vi "T7 CheckLength KAG.vi"(0 "Array":u8[](array[numeric])=[139, 242, 0, 160, 247, 0]) -> (1 "Array Output":u8[](array[numeric])=[139, 242, 0, 160, 247, 0], 2 "CheckLength Error":bool)   [LabVIEW 2015]
doc: "The LabJack T7 MODBUS Feedback Auto-Reponse Packet Protocol includes 2 Parameters that can be used to check packet integrity: (1) Length : # of bytes after \"Length\" parameter, (2) Number of samples. Though slightly redundant, one could also check the for the expected size of the entire Packet Byte Array. If any of the expected parameter values is not equal to the calculated length value, the CheckLength Error = TRUE.\n\n~~~~~~~~~~~~~~~~~~~~~~~~~~~~~~~~~~~\nMore Details:\n\nTransaction ID: The device echos this value. Use to match responses with commands.\nProtocol ID: Not used. Just pass 0.\nLength: The number of bytes after the \"Length\" parameter, per the Modbus spec.\nUnit ID: Not used. Pass 1 to fit with convention.\nFunctionn #: 3 (Read Multiple), 4 (Read One), 6 (Write One), 16 (Write Multiple) are standard Modbus \"holding\" functions. 76 (Feedback -- Multiple Reads & Writes in a single packet) is LJ custom MBFB function."
panel:
  out "Calculated # Bytes":i32
  out "Input # Bytes":i32
  out "Calculated # Samples":i32
  out "Input # Samples":i32
  out "Calculated Length":i32
  out "Input Length":i32
  # "Transaction ID"
  # "Protocol ID"
  # "MSB"
  # "Length"
  # "LSB"
  # "1 (Unit ID)"
  # "76 (Function)"
  # "MSB"
  # "# Samples"
  # "LSB"
  # "Backlog"
  # "Status Code"
  # "Additional Status Info"
  # "Stream Data"
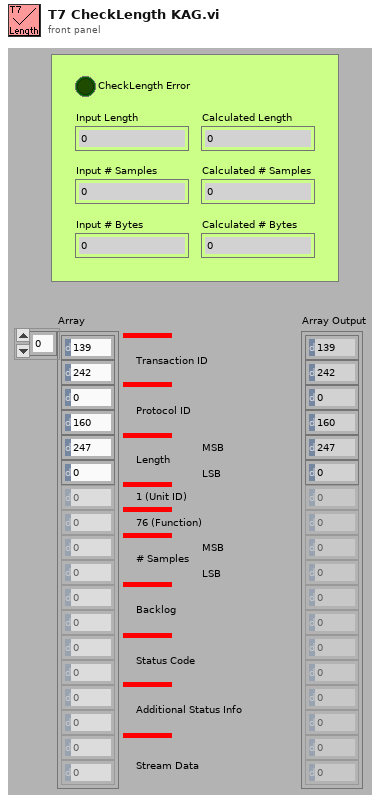
[diagram p1: front panel]
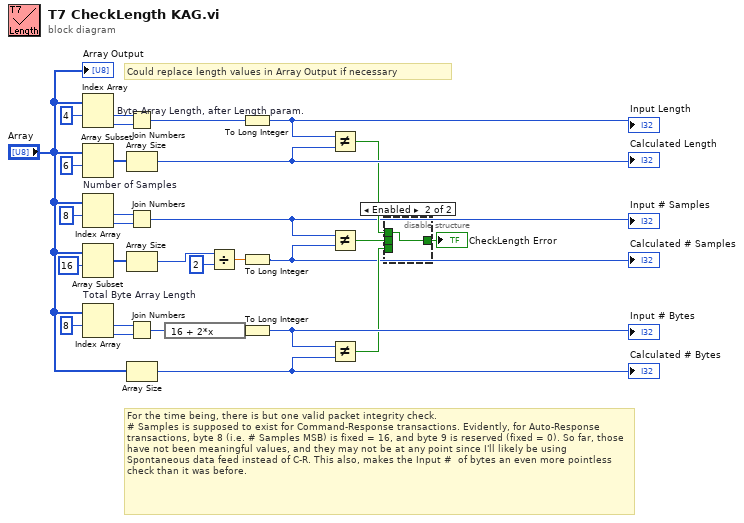
[diagram p0: block diagram]
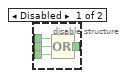
[diagram p2: hidden frame]
diagram:
  # "For the time being, there is but one valid packet integrity check.\n# Samples is supposed to exist for Command-Response transactions. Evidently, for Auto-Response transactions, byte 8 (i.e. # Samples MSB) is fixed = 16, and byte 9 is reserved (fixed = 0). So far, those have not been meaningful values, and they may not be at any point since I'll likely be using Spontaneous data feed instead of C-R. This also, makes the Input #  of bytes an even more pointless check than it was before."
  # "Could replace length values in Array Output if necessary"
  n1 = Index Array "Byte Array Length, after Length param."(array="Array", index #1=4 ("Index")) -> (element #1=w26:u8, element #2=w22:u8)  [unwired: 1 in]
  n2 = Array Subset(array="Array", index=6 ("Array Index")) -> (w27:u8[])  [unwired: 1 in]
  n3 = Index Array "Number of Samples"(array="Array", index #1=8 ("index")) -> (element #1=w21:u8, element #2=w20:u8)  [unwired: 1 in]
  n4 = Array Subset(array="Array", index=16 ("Array Index")) -> (w19:u8[])  [unwired: 1 in]
  n5 = Index Array "Total Byte Array Length"(array="Array", index #1=8 ("Index")) -> (element #1=w14:u8, element #2=w15:u8)  [unwired: 1 in]
  n6 = Join Numbers(hi=w26, lo=w22) -> ((hi.lo)=w25:u16)
  n7 = Array Size(array=w27) -> (size(s)=w24:i32)
  "Calculated Length" <- w24
  n8 = Join Numbers(hi=w21, lo=w20) -> ((hi.lo)=w1:u16)
  "Input # Samples" <- w1
  n9 = Array Size(array=w19) -> (size(s)=w3:i32)
  n10 = Join Numbers(hi=w14, lo=w15) -> ((hi.lo)=w6:u16)
  n11 = Array Size(array="Array") -> (size(s)=w4:i32)
  "Calculated # Bytes" <- w4
  n12 = expression code="16 + 2*x"(w6) -> (w5:u16)
  n13 = Divide(x=w3, y=u16 2) -> (x/y=w8:dbl)
  n14 = To Long Integer(number=w25) -> (32bit integer=w7:i32)
  "Input Length" <- w7
  n15 = To Long Integer(number=w8) -> (32bit integer=w2:i32)
  "Calculated # Samples" <- w2
  n16 = To Long Integer(number=w5) -> (32bit integer=w11:i32)
  "Input # Bytes" <- w11
  n17 = Not Equal?(x=w7, y=w24) -> (x != y?=w18:bool)
  n18 = Not Equal?(x=w1, y=w2) -> (x != y?=w17:bool)
  n19 = Not Equal?(x=w11, y=w4) -> (x != y?=w10:bool)
  n20 = disable-structure shown="Enabled" {
    disable-tunnel: w18 -> [w34 w35]
    disable-tunnel: w17 -> [w33 _]
    disable-tunnel: [w32 w35] -> w16
    disable-tunnel: w10 -> [w31 _]
    frame Disabled {
      n21 = Compound Arithmetic op=OR(w34, w33, w31) -> (w32:bool)
    }
    frame Enabled {
    }
  }
  "CheckLength Error" <- w16
  "Array Output" <- "Array"
